vi "Exercise 5.7.vi"() -> ()   [LabVIEW 2020]
panel:
  in  "Control Selection":dbl
  in  "Highlight":bool
  in  "Input 45":dbl
  in  "Input 44":dbl
  in  "Input 43":dbl
  in  "Input 42":dbl
  in  "Input 41":dbl
  in  "Input 40":dbl
  in  "Input 39":dbl
  in  "Input 38":dbl
  in  "Input 37":dbl
  in  "Input 36":dbl
  in  "Input 35":dbl
  in  "Input 34":dbl
  in  "Input 33":dbl
  in  "Input 32":dbl
  in  "Input 31":dbl
  in  "Input 30":dbl
  in  "Input 29":dbl
  in  "Input 28":dbl
  in  "Input 27":dbl
  in  "Input 26":dbl
  in  "Input 25":dbl
  in  "Input 24":dbl
  in  "Input 23":dbl
  in  "Input 22":dbl
  in  "Input 21":dbl
  in  "Input 20":dbl
  in  "Input 19":dbl
  in  "Input 18":dbl
  in  "Input 17":dbl
  in  "Input 16":dbl
  in  "Input 15":dbl
  in  "Input 14":dbl
  in  "Input 13":dbl
  in  "Input 12":dbl
  in  "Input 11":dbl
  in  "Input 10":dbl
  in  "Input 9":dbl
  in  "Input 8":dbl
  in  "Input 7":dbl
  in  "Input 6":dbl
  in  "Input 5":dbl
  in  "Input 4":dbl
  in  "Input 3":dbl
  in  "Input 2":dbl
  in  "Input 1":dbl
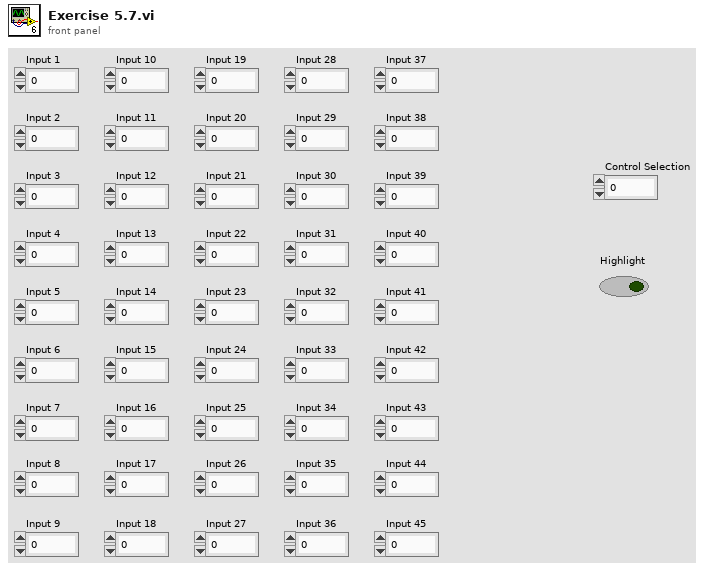
[diagram p1: front panel]
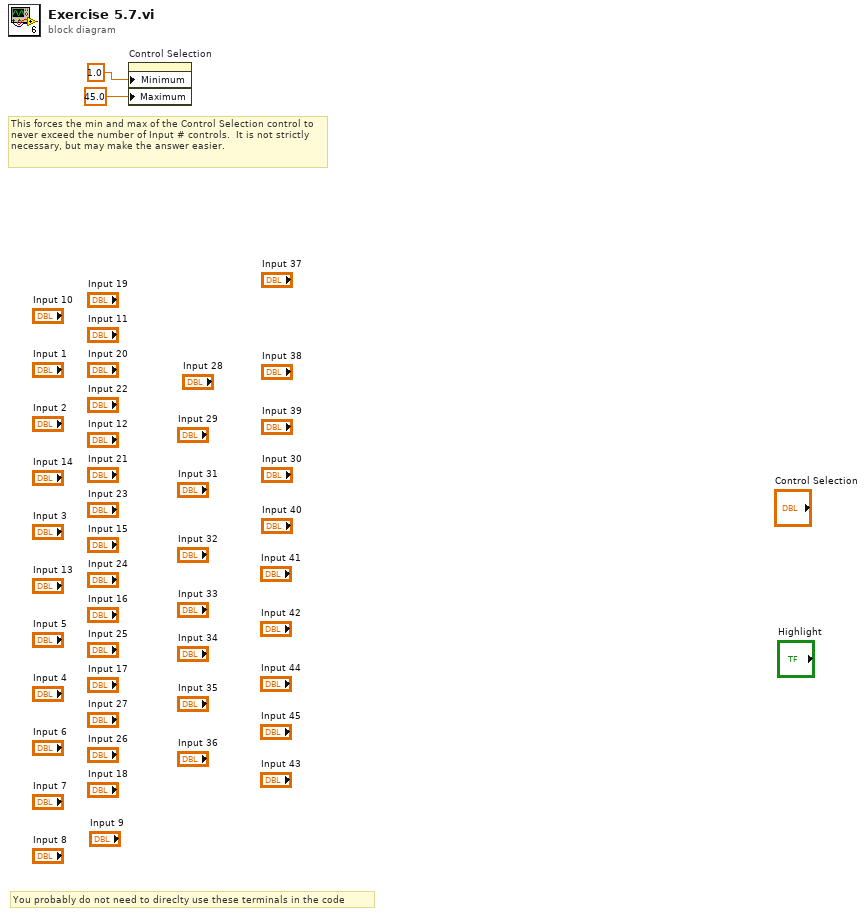
[diagram p0: block diagram]
diagram:
  # "This forces the min and max of the Control Selection control to never exceed the number of Input # controls.  It is not strictly necessary, but may make the answer easier."
  # "You probably do not need to direclty use these terminals in the code"
  n1 = property on="Control Selection" class="DigNum (strict)"("Minimum"=1.0 ("Data Entry Limits:Minimum"), "Maximum"=45.0 ("Data Entry Limits:Maximum")) -> ()  [unwired: 2 in, 2 out]
